vi "constructor.vi"(10 "Beverage.lvclass":refnum<class "Beverage.lvclass">, 11 "Milk in":refnum<class "Milk.lvclass">) -> (3 "Milk out":refnum<class "Milk.lvclass">)   [LabVIEW 2020, in "Milk.lvclass"]
uses:
  Milk.lvclass
  Beverage.lvclass
  Milk.lvclass/Milk.ctl
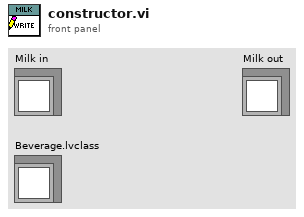
[diagram p1: front panel]
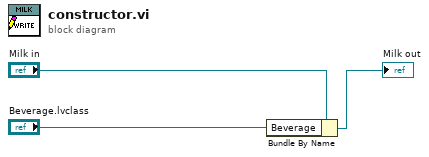
[diagram p0: block diagram]
diagram:
  n1 = Bundle By Name(cluster="Milk in", "Beverage"="Beverage.lvclass") -> (→"Milk out":refnum<class "Milk.lvclass">)
